vi "INit6009.vi"(7 "Range":dbl[](array[numeric]), 8 "error in (no error)":errorcluster, 9 "ChannelEnable":T1[](array[typedef]), 10 "DAQmx Device Name":tag="Dev2", 11 "Trigger":bool) -> (0 "error out":errorcluster, 2 "DAQmx Device Name out":tag="Dev2", 3 "Refnum out":refnum<k21>)   [LabVIEW 2011]
uses:
  OnOffTypeDef.ctl
panel:
  out "AI.PhysicalChans":tag[](array[tag])
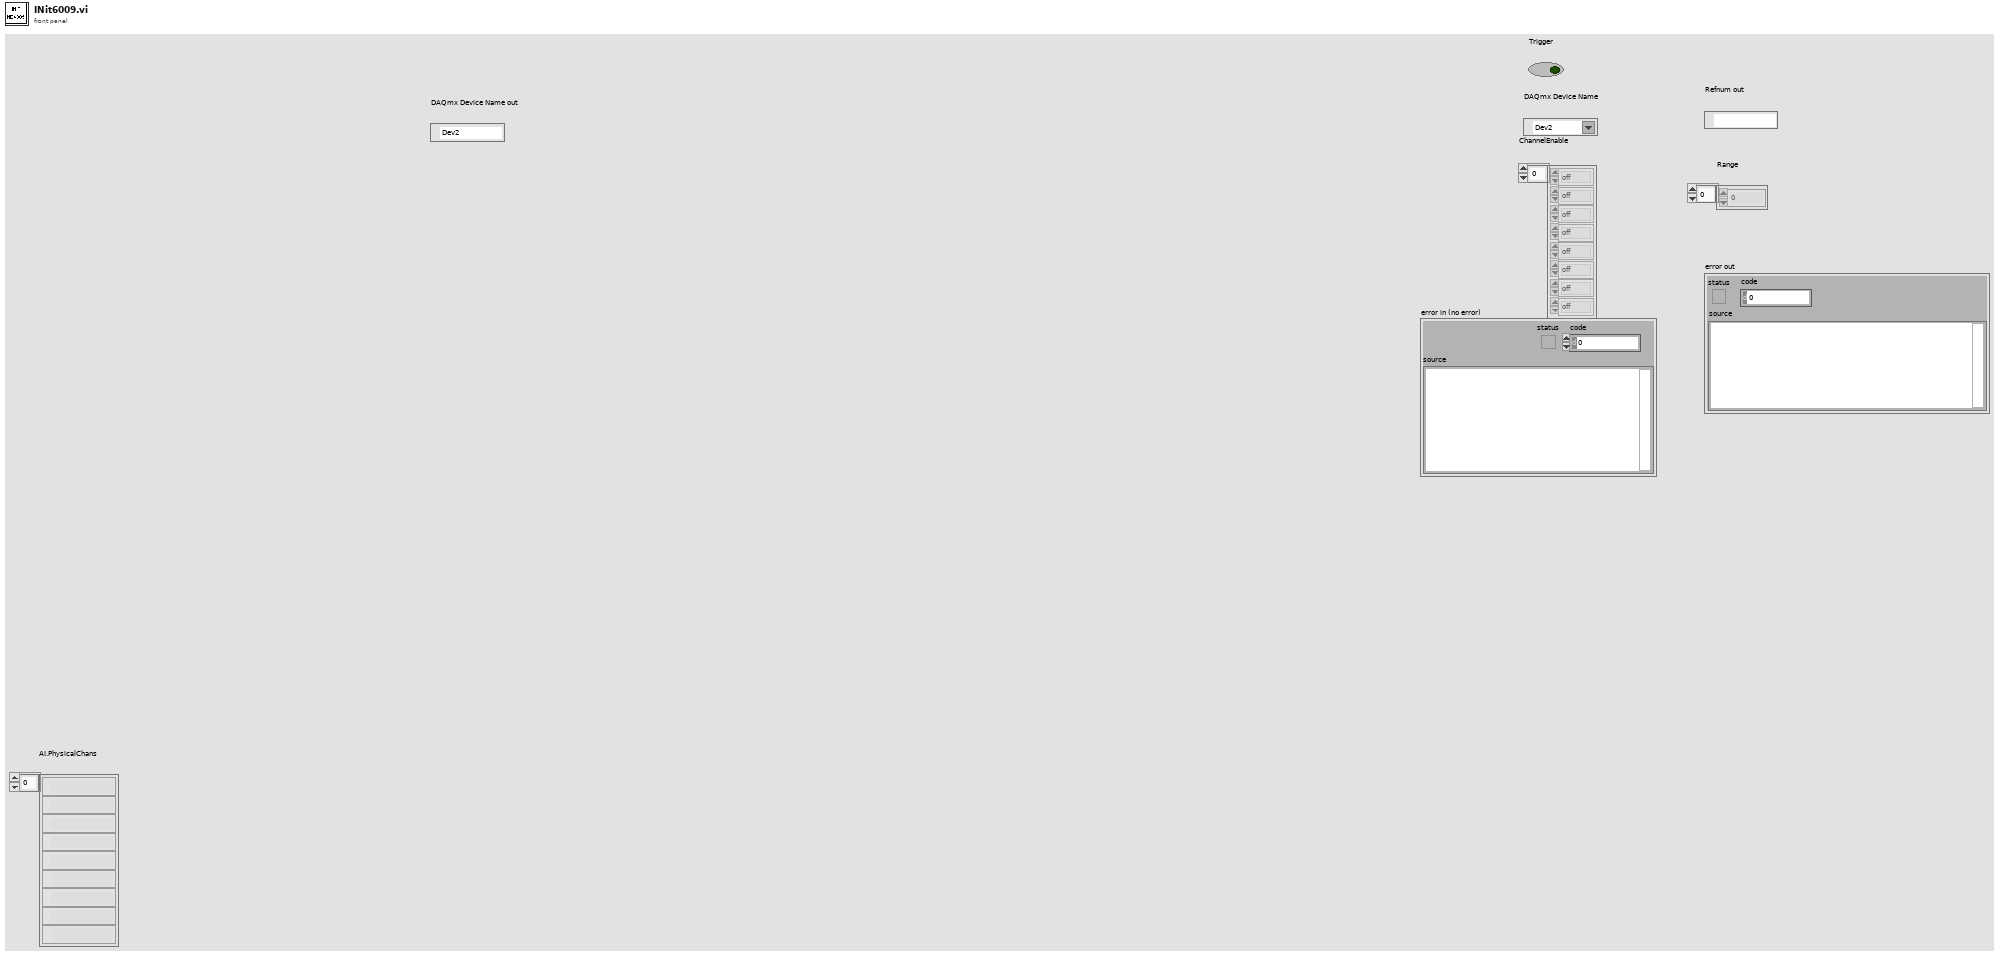
[diagram p1: front panel]
types:
  T1 = typedef "OnOffTypeDef.ctl" = enum16{"off", "on"}
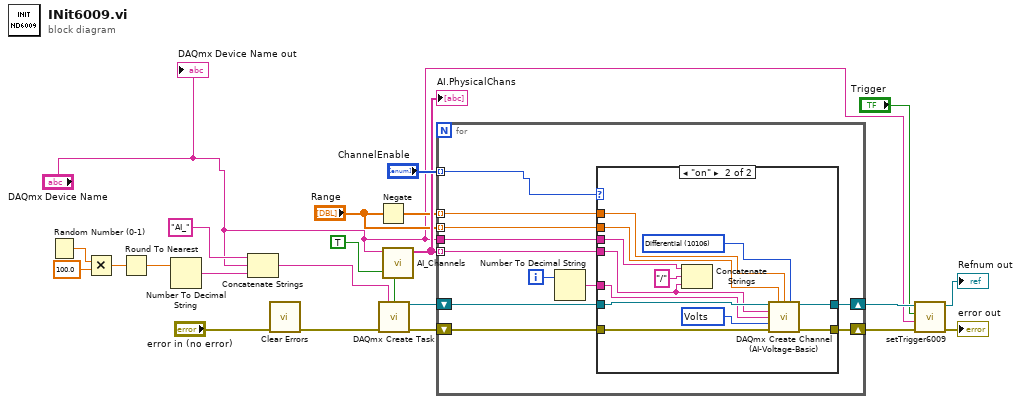
[diagram p0: block diagram]
diagram:
  n1 = Random Number (0-1)() -> (number: 0 to 1=w13:dbl)
  n2 = Multiply(x=w13, y=100.0) -> (x*y=w11:dbl)
  n3 = Round To Nearest(number=w11) -> (nearest integer value=w10:dbl)
  n4 = Number To Decimal String(number=w10) -> (decimal integer string=w9:string)  [unwired: 1 in]
  n5 = Concatenate Strings("AI_", "DAQmx Device Name", w9) -> (w14:string)
  n6 = call "Clear Errors.vi"("error in (no error)"="error in (no error)") -> ("error out"=w3:errorcluster)  [unwired: 6 in]
  n7 = Negate(x="Range") -> (-x=w5:dbl[])
  n8 = call "DAQmx Create Task.vi"("new task name"=w14, "auto cleanup"=TRUE, "error in"=w3) -> ("task out"=w17:refnum<k21>, "error out"=w15:errorcluster)  [unwired: 11 in]
  n9 = call "AI_Channels.vi"("DAQmx Device Name"="DAQmx Device Name") -> ("Array"=w7:tag[])  [unwired: 9 in, 1 out]
  "AI.PhysicalChans" <- w7
  n10 = for {
    tunnel: "DAQmx Device Name" -> [w33]
    shift-right: [w31] -> w22
    shift-left: w17 -> [w32]
    shift-right: [w30] -> w18
    shift-left: w15 -> [w29]
    tunnel: "ChannelEnable" -> [w24] mode=indexing
    tunnel: w5 -> [w28] mode=indexing
    tunnel: "Range" -> [w27] mode=indexing
    tunnel: w7 -> [w26] mode=indexing
    i -> [w23]
    n11 = Number To Decimal String(number=w23) -> (decimal integer string=w25:string)  [unwired: 1 in]
    n12 = case shown="\"on\"" w24 {
      tunnel: w33 -> [_ w45]
      tunnel: w32 -> [w35 w44]
      tunnel: [w35 w43] -> w31
      tunnel: [w34 w41] -> w30
      tunnel: w29 -> [w34 w40]
      tunnel: w28 -> [_ w39]
      tunnel: w27 -> [_ w38]
      tunnel: w26 -> [_ w37]
      tunnel: w25 -> [_ w36]
      frame "off", Default {
      }
      frame "on" {
        w42 = 10348 items=["Volts"=10348, "From Custom Scale"=10065] ("units")
        w47 = 10106 items=["default"=-1, "RSE"=10083, "NRSE"=10078, "Differential"=10106, "Pseudodifferential"=12529] ("input terminal configuration")
        n13 = Concatenate Strings(w45, "/" ("string"), w37) -> ()  [unwired: 1 out]
        n14 = call "DAQmx Create Channel (AI-Voltage-Basic).vi"("task in"=w44, "maximum value"=w38, "minimum value"=w39, "input terminal configuration"=w47, "physical channels"=w37, "name to assign"=w36, "units"=w42, "error in"=w40) -> ("task out"=w43:refnum<k21>, "error out"=w41:errorcluster)  [unwired: 6 in]
      }
    }
  }
  n15 = call "setTrigger6009.vi"("error in (no error)"=w18, "Device Name in"="DAQmx Device Name", "Trigger"="Trigger", "Refnum in"=w22) -> ("error out"=→"error out":errorcluster, "Refnum out"=→"Refnum out":refnum<k21>)  [unwired: 5 in, 1 out]
  "DAQmx Device Name out" <- "DAQmx Device Name"
